vi "Set Highlighted.vi"(8 "error in (no error)":errorcluster, 10 "Highlighted":bool, 11 "GWebAppArrayPanel in":refnum<class "GWebAppArrayPanel.lvclass">) -> (0 "error out":errorcluster, 3 "GWebAppArrayPanel out":refnum<class "GWebAppArrayPanel.lvclass">)   [LabVIEW 2020, in "PicoG-App.lvlib" / "GWebAppArrayPanel.lvclass"]
uses:
  GWebAppArrayPanel.lvclass
  GWebAppArrayPanel.lvclass/GWebAppArrayPanel.ctl
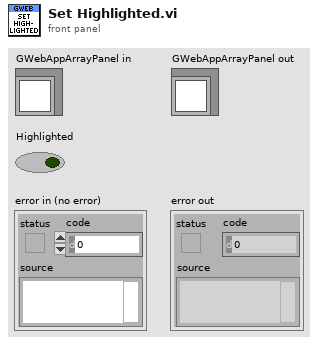
[diagram p1: front panel]
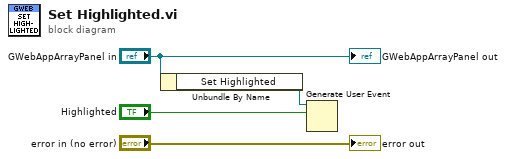
[diagram p0: block diagram]
diagram:
  n1 = Unbundle By Name("GWebAppArrayPanel in") -> ("Set Highlighted"=w2:refnum<user-event>)
  n2 = Generate User Event(user event=w2, event data cluster="Highlighted") -> ()  [unwired: 2 in, 2 out]
  "error out" <- "error in (no error)"
  "GWebAppArrayPanel out" <- "GWebAppArrayPanel in"
